vi "Qrcode Sort.vi"() -> ()   [LabVIEW 2019]
uses:
  <vilib>/userDefined/High Color/IMAQdx.ctl
  <vilib>/vision/driver/NI_Vision_Acquisition_Software.lvlib
  <vilib>/vision/NI_Vision_Development_Module.lvlib
panel:
  out "Index ke-":dbl
  out "Blue":bool
  out "Green":bool
  out "Yellow":bool
  out "Codes":string[](array[string])
  in  "Array":T1(array[cluster])
  out "Enum":enum16{"scan", "execute"}(ring)
  out "Numeric":dbl
  out "element":string
  out "element 2":string
  out "element 3":string
  out "Array 2":string[](array[string])
  out "Found?":bool
  out "Image":T2(plugin-control)
  out "Data":string
  in  "Session In":T3
  out "sorted array":string[](array[string])
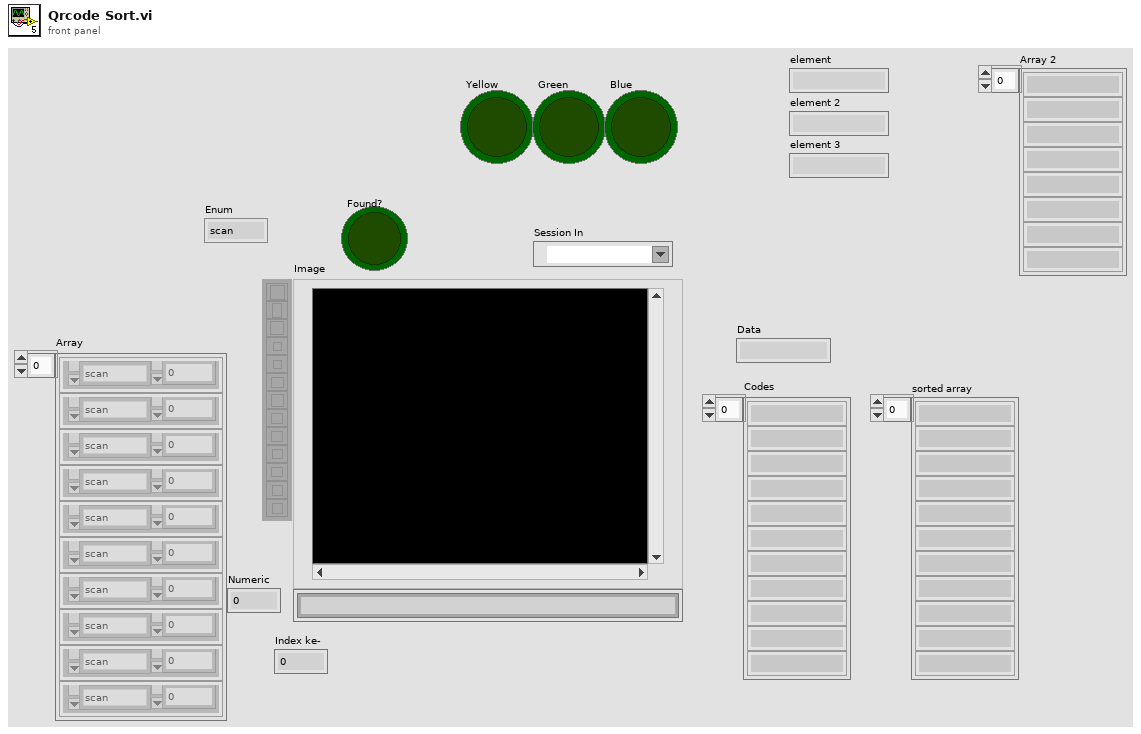
[diagram p1: front panel]
types:
  T1 = cluster{"Enum":enum16{"scan", "execute"}, "Numeric":dbl}[]
  T2 = typedef "IMAQ Image.ctl" = refnum<image>
  T3 = typedef "IMAQdx.ctl" = refnum<k21>
  T4 = typedef "Image Type" = u32
  T5 = typedef "QR Code Report.ctl" = cluster{"Found?":bool, "Data":string, "Bounding Box":cluster{"x":sgl, "y":sgl}[], "Errors Corrected":u32, "Dimensions (Rows/Cols)":u32, "Version":u32, "QR Model":T6, "Stream Mode":T7, "Barcode Polarity":T8, "Mirrored?":bool, "Append Stream Position":u32, "Size of Append Stream":u32, "First EAN-128 ID":i32, "First Alternate Language ID":i32, "Append Stream ID":u32, "Minimum Edge Strength":u32, "Demodulation Mode":T9, "Cell Sample Size":T10, "Cell Filter Mode":T11}
  T6 = typedef "QR Code Model Type.ctl" = i32
  T7 = typedef "QR Code Stream Mode Type.ctl" = i32
  T8 = typedef "Data Matrix Polarity.ctl" = i32
  T9 = typedef "Demodulation Mode.ctl" = i32
  T10 = typedef "Cell Sample Size.ctl" = i32
  T11 = typedef "Cell Filter Mode.ctl" = i32
  T12 = cluster{"Enum":enum16{"scan", "execute"}, "Numeric":dbl}
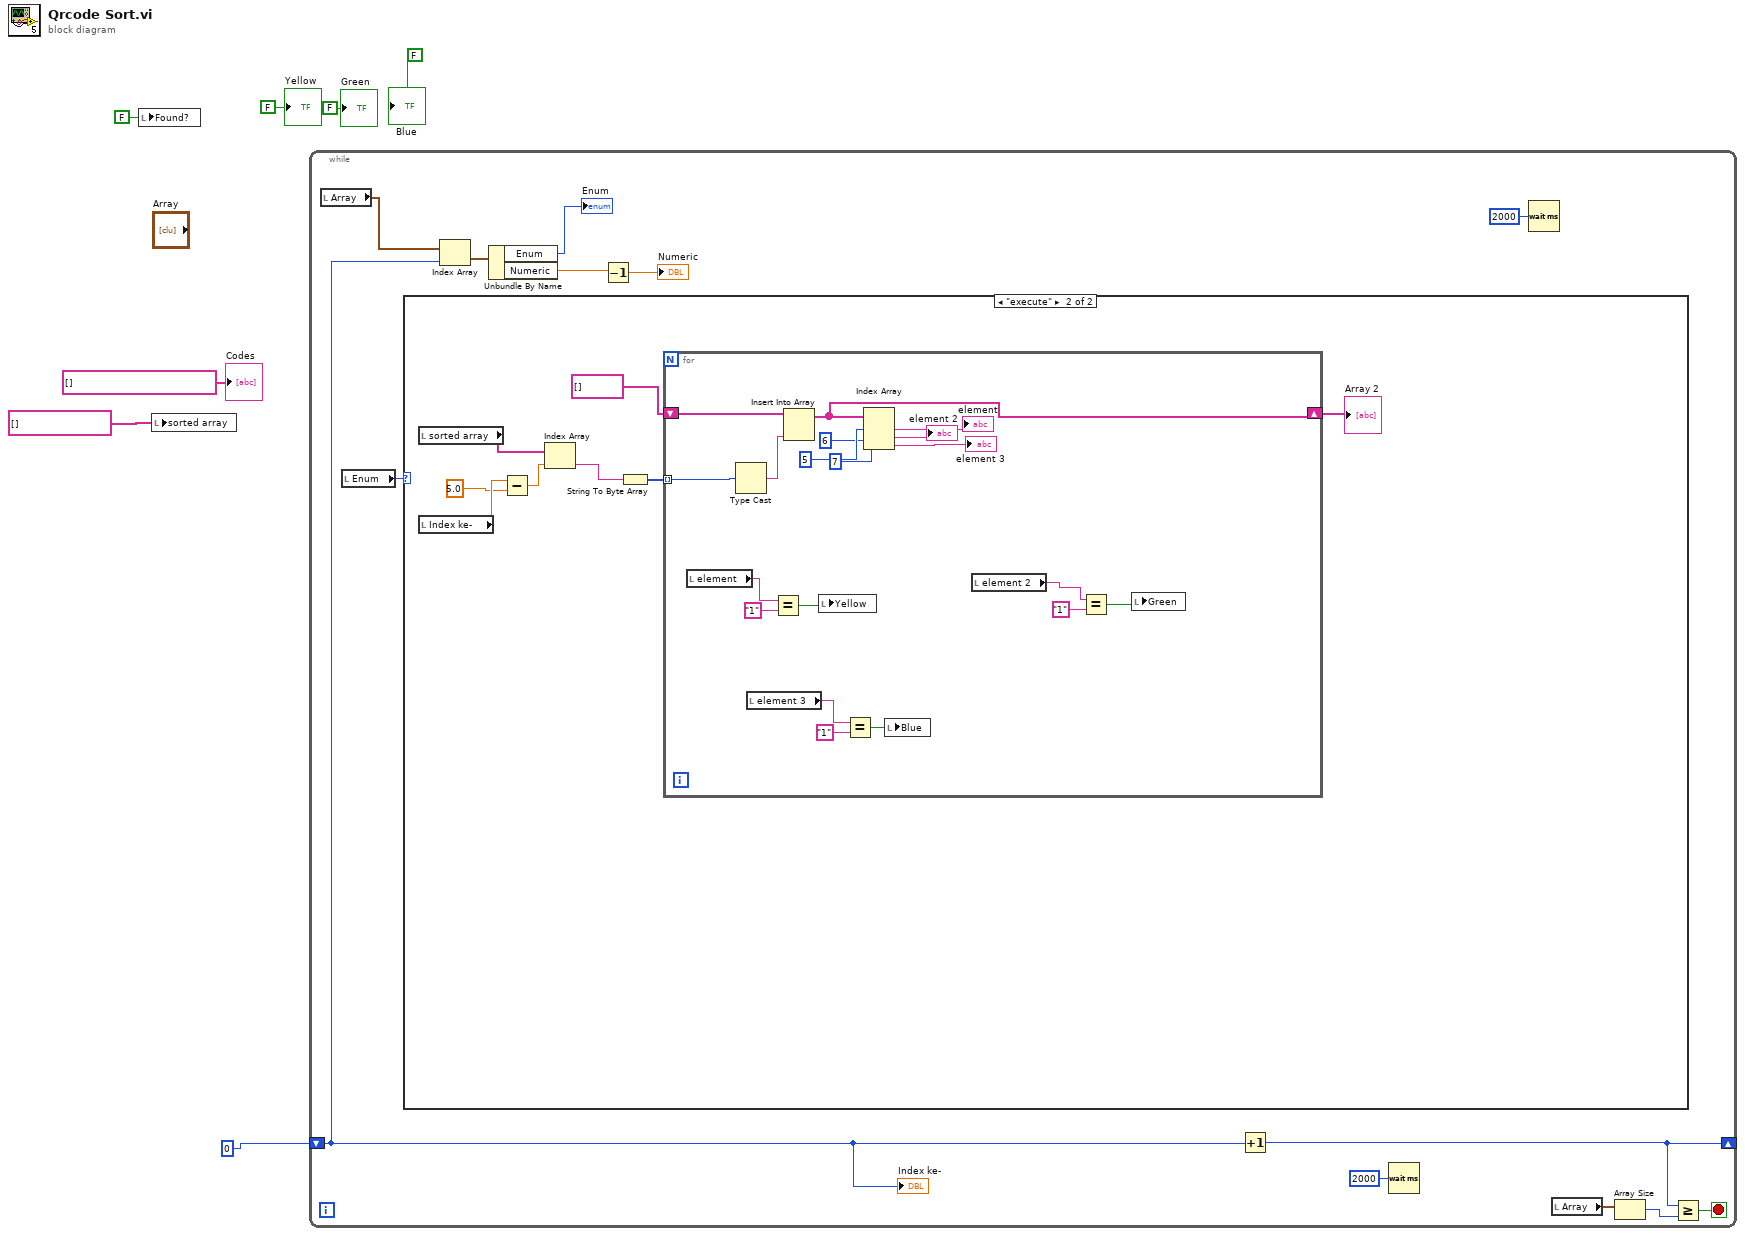
[diagram p0: block diagram]
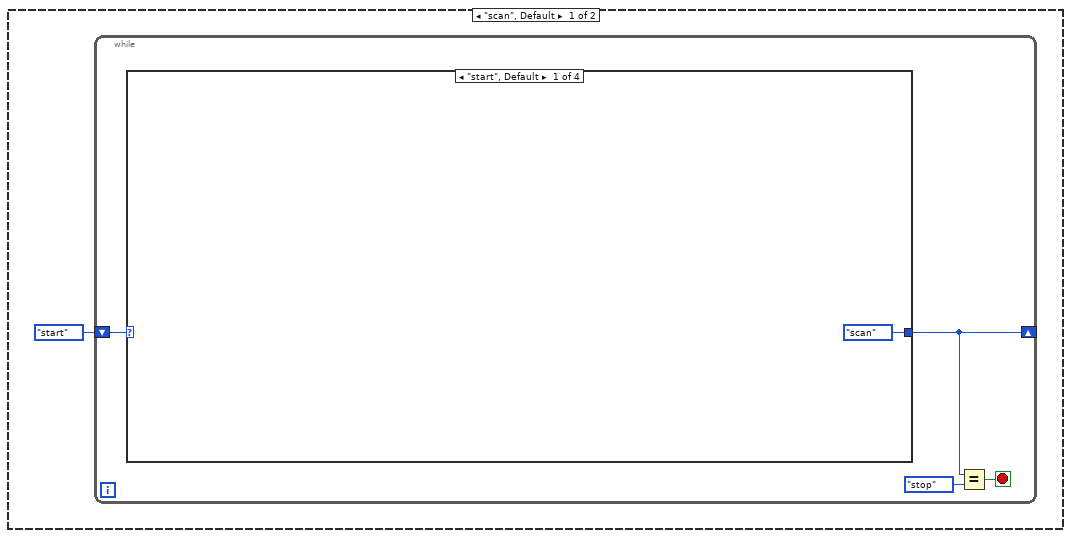
[diagram p2: hidden frame]
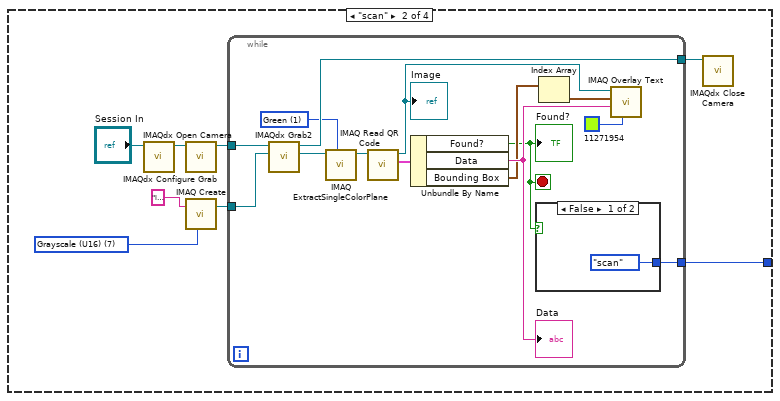
[diagram p3: hidden frame]
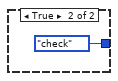
[diagram p4: hidden frame]
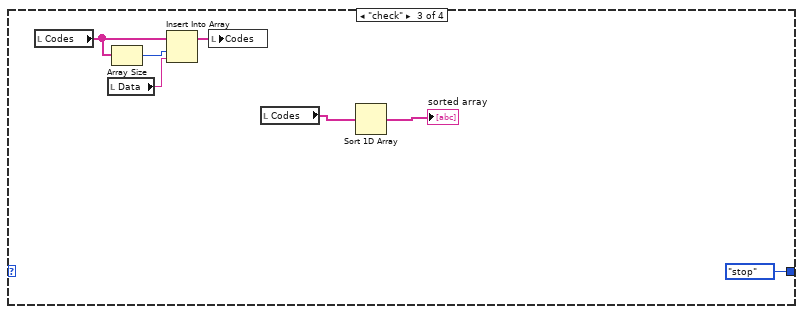
[diagram p5: hidden frame]
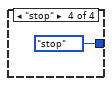
[diagram p6: hidden frame]
diagram:
  n1 = local write "Found?"(FALSE ("Found?")) -> ()
  n2 = local write "sorted array"(string[] [] ("sorted array")) -> ()
  n3 = while {
    shift-right: [w18] -> _
    shift-left: 0 -> [w8]
    stop <- w19 stop-if-true
    n4 = local read "Array"() -> (w17:T1)
    n5 = local read "Enum"() -> (w12:enum16{"scan", "execute"})
    n6 = case shown="\"execute\"" w12 {
      frame "scan", Default {
        n7 = while {
          shift-right: [w22] -> _
          shift-left: enum16{"start", "scan", "check", "stop"}."start" -> [w25]
          stop <- w23 stop-if-true
          n8 = case shown="\"start\", Default" w25 {
            tunnel: [enum16{"start", "scan", "check", "stop"}."scan" w27 enum16{"start", "scan", "check", "stop"}."stop" enum16{"start", "scan", "check", "stop"}."stop"] -> w22
            frame "start", Default {
            }
            frame "scan" {
              w29 = T4 7 items=["Grayscale (U8)", "Grayscale (I16)", "Grayscale (SGL)", "Complex (CSG)", "RGB (U32)", "HSL (U32)", "RGB (U64)", "Grayscale (U16)"] ("Image Type")
              n9 = call <vilib>:"IMAQdx Open Camera.vi"("Session In"="Session In") -> ("Session Out"=w33:T3)  [unwired: 9 in, 1 out]
              n10 = call <vilib>:"IMAQdx Configure Grab.vi"("Session In"=w33) -> ("Session Out"=w31:T3)  [unwired: 9 in, 1 out]
              n11 = call "IMAQ Create"("Image Name"="img", "Image Type"=w29) -> ("New Image"=w28:T2)  [unwired: 3 in, 1 out]
              n12 = while {
                tunnel: [w48] -> w32
                tunnel: w31 -> [w47]
                tunnel: w28 -> [w46]
                tunnel: [w35] -> w27
                stop <- w36 stop-if-true
                w43 = 1 items=["Red", "Green", "Blue", "Hue", "Saturation", "Luminance", "Value", "Intensity"] ("Color Plane")
                n13 = call <vilib>:"IMAQdx Grab2.vi"("Image In"=w46, "Session In"=w47) -> ("Image Out"=w45:T2, "Session Out"=w48:T3)  [unwired: 6 in, 2 out]
                n14 = call "IMAQ ExtractSingleColorPlane"("Color Plane"=w43, "Image Src"=w45) -> ("Image Dst Out"=w44:T2)  [unwired: 8 in, 1 out]
                n15 = call "IMAQ Read QR Code"("Image"=w44) -> ("QR Code Report"=w42:T5, "Image (duplicate)"=w37:T2)  [unwired: 7 in, 2 out]
                "Image" <- w37
                n16 = Unbundle By Name(w42) -> ("Found?"=w36:bool, "Data"=w40:string, "Bounding Box"=w38:cluster{"x":sgl, "y":sgl}[])
                "Found?" <- w36
                "Data" <- w40
                n17 = case shown="False" w36 {
                  tunnel: [enum16{"start", "scan", "check", "stop"}."scan" enum16{"start", "scan", "check", "stop"}."check"] -> w35
                  frame False {
                  }
                  frame True {
                  }
                }
                n18 = Index Array(array=w38) -> (element=w41:cluster{"x":sgl, "y":sgl})  [unwired: 1 in]
                n19 = call "IMAQ Overlay Text"("Text Color (black)"=u32 11271954, "String"=w40, "Origin"=w41, "Image"=w37) -> ()  [unwired: 6 in, 2 out]
              }
              n20 = call <vilib>:"IMAQdx Close Camera.vi"("Session In"=w32) -> ()  [unwired: 10 in, 1 out]
            }
            frame "check" {
              n21 = local read "Codes"() -> (w57:string[])
              n22 = local read "Data"() -> (w55:string)
              n23 = Array Size(array=w57) -> (size(s)=w56:i32)
              n24 = Insert Into Array(array=w57, index=w56, new element=w55) -> (w54:string[])
              n25 = local write "Codes"(w54) -> ()
              n26 = local read "Codes"() -> (w51:string[])
              n27 = Sort 1D Array(array=w51) -> (sorted array=→"sorted array":string[])
            }
            frame "stop" {
            }
          }
          n28 = Equal?(x=w22, y=enum16{"start", "scan", "check", "stop"}."stop") -> (x = y?=w23:bool)
        }
      }
      frame "execute" {
        n29 = local read "sorted array"() -> (w66:string[])
        n30 = local read "Index ke-"() -> (w60:dbl)
        n31 = Subtract(x=w60, y=5.0) -> (x-y=w61:dbl)
        n32 = Index Array(array=w66, index=w61) -> (element=w65:string)
        n33 = String To Byte Array(string=w65) -> (unsigned byte array=w64:u8[])
        n34 = for {
          tunnel: w64 -> [w85] mode=indexing
          shift-right: [w76] -> w62
          shift-left: string[] [] -> [w84]
          n35 = local read "element"() -> (w75:string)
          n36 = Type Cast(x=w85) -> (*(type *) &x=w83:string)  [unwired: 1 in]
          n37 = local read "element 3"() -> (w71:string)
          n38 = Equal?(x=w75, y="1") -> (x = y?=w69:bool)
          n39 = Insert Into Array(array=w84, new element=w83) -> (w76:string[])  [unwired: 1 in]
          n40 = local write "Yellow"(w69) -> ()
          n41 = Equal?(x=w71, y="1") -> (x = y?=w68:bool)
          n42 = Index Array(array=w76, index #1=5 ("index"), index #2=6 ("index"), index #3=7 ("index")) -> (element #1=→"element":string, element #2=→"element 2":string, element #3=→"element 3":string)
          n43 = local write "Blue"(w68) -> ()
          n44 = local read "element 2"() -> (w73:string)
          n45 = Equal?(x=w73, y="1") -> (x = y?=w67:bool)
          n46 = local write "Green"(w67) -> ()
        }
        "Array 2" <- w62
      }
    }
    n47 = Index Array(array=w17, index=w8) -> (element=w14:T12)
    n48 = Unbundle By Name(w14) -> ("Enum"=→"Enum":enum16{"scan", "execute"}, "Numeric"=w10:dbl)
    n49 = Decrement(x=w10) -> (x-1=→"Numeric":dbl)
    n50 = Increment(x=w8) -> (x+1=w18:i32)
    n51 = Wait (ms)(milliseconds to wait=u32 2000) -> ()  [unwired: 1 out]
    n52 = Wait (ms)(milliseconds to wait=u32 2000) -> ()  [unwired: 1 out]
    n53 = local read "Array"() -> (w15:T1)
    n54 = Array Size(array=w15) -> (size(s)=w16:i32)
    n55 = Greater Or Equal?(x=w18, y=w16) -> (x >= y?=w19:bool)
    "Index ke-" <- w8
  }
  "Codes" <- string[] [] ("Array 2")
  "Yellow" <- FALSE ("Yellow")
  "Green" <- FALSE ("Green")
  "Blue" <- FALSE ("Blue")
